vi "read or write files.vi"() -> ()   [LabVIEW 2018]
panel:
  out "text 2":string
  in  "text":string
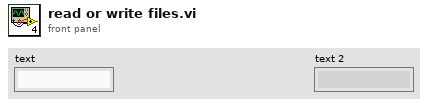
[diagram p1: front panel]
types:
  T1 = enum16{"open", "replace", "create", "open or create", "replace or create", "replace or create with confirmation"}
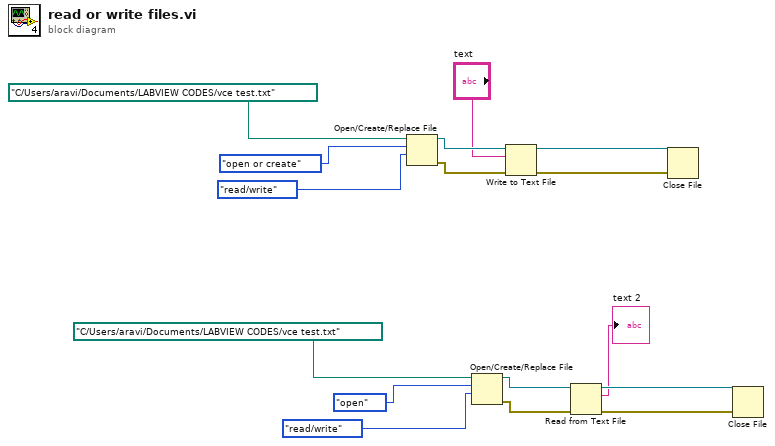
[diagram p0: block diagram]
diagram:
  n1 = Open/Create/Replace File(file path (use dialog)=path "C:/Users/aravi/Documents/LABVIEW CODES/vce test.txt", operation (0:open)=T1."open or create", access (0:read/write)=enum16{"read/write", "read-only", "write-only"}."read/write") -> (refnum out=w13:refnum<file>, error out=w12:errorcluster)  [unwired: 3 in, 1 out]
  n2 = Open/Create/Replace File(file path (use dialog)=path "C:/Users/aravi/Documents/LABVIEW CODES/vce test.txt", operation (0:open)=T1."open", access (0:read/write)=enum16{"read/write", "read-only", "write-only"}."read/write") -> (refnum out=w5:refnum<file>, error out=w4:errorcluster)  [unwired: 3 in, 1 out]
  n3 = Write to Text File(file (use dialog)=w13, text="text", error in=w12) -> (refnum out=w10:refnum<file>, error out=w11:errorcluster)  [unwired: 1 in, 1 out]
  n4 = Read from Text File(file (use dialog)=w5, error in=w4) -> (refnum out=w2:refnum<file>, text=→"text 2":string, error out=w3:errorcluster)  [unwired: 2 in, 1 out]
  n5 = Close File(refnum=w10, error in=w11) -> ()  [unwired: 2 out]
  n6 = Close File(refnum=w2, error in=w3) -> ()  [unwired: 2 out]
